vi "PH_Stepmotor_BaseClass.PC set Position.vi"(0 "i ref in":refnum<vi>, 1 "axis":i32=-1, 2 "Position to set":i32, 3 "Set?":bool, 5 "error in (no error)":errorcluster) -> (14 "i ref out":refnum<vi>, 16 "ok?":bool, 19 "error out":errorcluster)   [LabVIEW 2014, in "PH_Stepmotor_BaseClass.lvlib"]
doc: "This VI stores the position in own attributes and sets a flag."
uses:
  PH_Stepmotor_BaseClass.lvlib
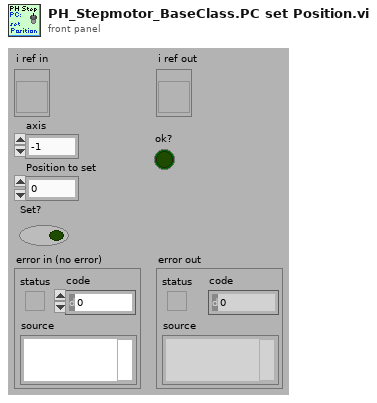
[diagram p1: front panel]
types:
  T1 = typedef "PH_Stepmotor_BaseClass.lvlib/PH_Stepmotor_BaseClass.Axis Attributes.ctl" = cluster{"Settings":T2, "Endswitch?":bool, "DIM Service IDs":T4, "Activity":T5, "Configured?":bool, "Position":cluster{"Current":i32, "Target":i32}, "Position to set":cluster{"New?":bool, "Wanted":i32}, "Stop?":bool, "Reset?":bool, "Move?":bool, "Nothing connected?":bool}
  T2 = typedef "PH_Stepmotor_BaseClass.lvlib/PH_Stepmotor_BaseClass.Axis Settings.ctl" = cluster{"Sign change":bool, "Width":dbl, "Calibration":dbl, "Unit":string, "Motor Type":T3, "Unit Width":string, "Unit CF":string}
  T3 = typedef "PH_Stepmotor_BaseClass.lvlib/PH_Stepmotor_BaseClass.Motor Type.ctl" = enum16{"Unspecific", "OWIS 49.120.2633", "OWIS 49.060.1033", "OWIS 43.040.2558", "Diamond Motion 2200 series", "OWIS 49.120.266B.MV6", "Calorimeter", "Linear Stage 1", "MICOS VT-80", "MICOS VT-80 S", "Standa Rotstage nt0.95A", "PUF RA 320.200", "PUF RA 800.200", "PUF RA 800.400", "PUF RA 400.50", "1324.nn.800.50", "1324.n9c.800.50", "1324.nn.320.200", "1324.nn.400.200", "1324.nn.800.200", "1324.nn.400.50", "1324.8c9c.800.50", "1324.8c9c.400.200"}
  T4 = typedef "PH_Stepmotor_BaseClass.lvlib/PH_Stepmotor_BaseClass.Axis DIM Service IDs.ctl" = cluster{"Settings":i32, "Information":i32}
  T5 = typedef "PH_Stepmotor_BaseClass.lvlib/PH_Stepmotor_BaseClass.Axis Activity.ctl" = enum16{"No Information", "stopped", "running", "Failure", "Alarm", "stopped at backward ES", "stopped at foreward ES"}
  T6 = typedef "PH_Stepmotor_BaseClass.lvlib/PH_Stepmotor_BaseClass.i attribute.ctl" = cluster{"Device Error":errorcluster, "Axes PSDB Thread":cluster{"Ref":refnum<vi>, "Q-Ref":refnum<queue>, "Data Status":T7}, "Axes":T1[], "Axes PSDB Infos":cluster{"GUI Name":string, "PSDB Instance ID":i32, "PSDB Status Service ID":i32, "Axis":i32, "Class":string}[], "GUI Refs":T8}
  T7 = typedef "PH_PSDBWriter.lvlib/PH_PSDBWriter.Data Status.ctl" = i16
  T8 = typedef "PH_Stepmotor_BaseClass.lvlib/PH_Stepmotor_BaseClass.GUI Refs.ctl" = cluster{"Axes Configuration":refnum<vi>, "Device Error":refnum<vi>, "Axes PSDB Infos":refnum<vi>}
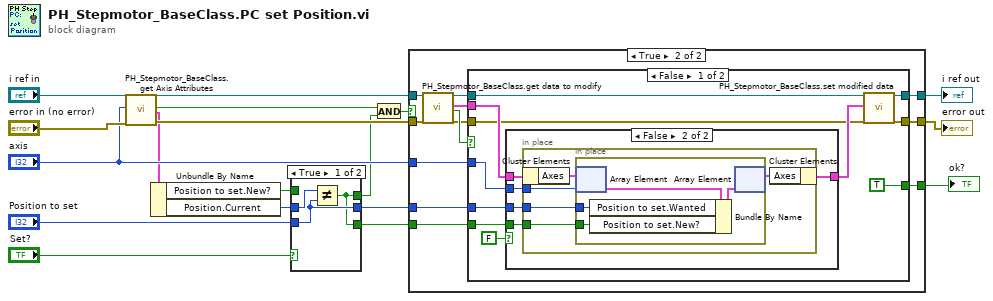
[diagram p0: block diagram]
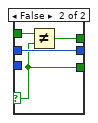
[diagram p2: hidden frame]
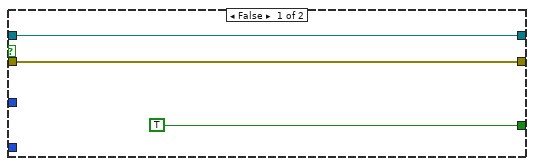
[diagram p3: hidden frame]
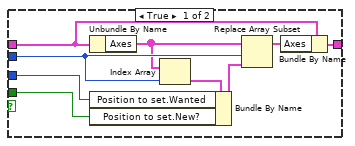
[diagram p4: hidden frame]
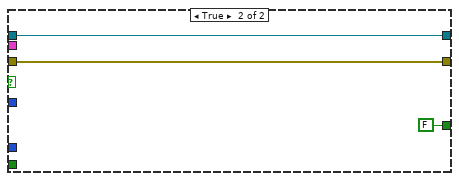
[diagram p5: hidden frame]
diagram:
  n1 = call "PH_Stepmotor_BaseClass.get Axis Attributes.vi"("VI in"="i ref in", "Axis"="axis", "error in (no error)"="error in (no error)") -> ("VI out"=w13:refnum<vi>, "Axis found?"=w11:bool, "Axis Attributes"=w8:T1, "error out"=w15:errorcluster)  [unwired: 13 in]
  n2 = Unbundle By Name(w8) -> ("Position to set.New?"=w3:bool, "Position.Current"=w7:i32)
  n3 = case shown="True" "Set?" {
    selector: "Set?" -> [_ w22]
    tunnel: [w19 w24] -> w2
    tunnel: "Position to set" -> [w20 _]
    tunnel: w7 -> [w21 w23]
    tunnel: [w20 w23] -> w5
    tunnel: w3 -> [_ w25]
    tunnel: [w19 w22] -> w1
    frame True {
      n4 = Not Equal?(x=w21, y=w20) -> (x != y?=w19:bool)
    }
    frame False {
      n5 = Not Equal?(x=w25, y=w22) -> (x != y?=w24:bool)
    }
  }
  n6 = And(x=w11, y=w2) -> (x .and. y?=w10:bool)
  n7 = case shown="True" w10 {
    tunnel: [w28 w36] -> w17
    tunnel: [w27 w35] -> w16
    tunnel: w15 -> [w27 w34]
    tunnel: w13 -> [w28 w33]
    tunnel: "axis" -> [_ w32]
    tunnel: w5 -> [_ w31]
    tunnel: w1 -> [_ w30]
    tunnel: [TRUE w29] -> w4
    frame False {
    }
    frame True {
      n8 = call "PH_Stepmotor_BaseClass.get data to modify.vi"("i ref in"=w33, "error in (no error)"=w34) -> ("i ref out"=w38:refnum<vi>, "i attribute"=w37:T6, "timed out"=w40:bool, "error out"=w39:errorcluster)  [unwired: 14 in]
      n9 = case shown="False" w40 {
        tunnel: [w51 w77] -> w35
        tunnel: w39 -> [w44 w77]
        tunnel: [w50 w76] -> w36
        tunnel: w38 -> [w47 w76]
        tunnel: w37 -> [w49 _]
        tunnel: w32 -> [w46 _]
        tunnel: w31 -> [w45 _]
        tunnel: w30 -> [w42 _]
        tunnel: [TRUE FALSE] -> w29
        frame False {
          n10 = case shown="False" FALSE {
            tunnel: w49 -> [w53 w62]
            tunnel: [w60 w61] -> w48
            tunnel: w46 -> [w58 w65]
            tunnel: w45 -> [w57 w64]
            tunnel: w42 -> [w52 w63]
            frame True {
              n11 = Unbundle By Name(w53) -> ("Axes"=w55:T1[])
              n12 = Index Array(array=w55, index=w58) -> (element=w54:T1)
              n13 = Bundle By Name(cluster=w54, "Position to set.Wanted"=w57, "Position to set.New?"=w52) -> (w56:T1)
              n14 = Replace Array Subset(array=w55, new element=w56, index=w58) -> (w59:T1[])
              n15 = Bundle By Name(cluster=w53, "Axes"=w59) -> (w60:T6)
            }
            frame False {
              n16 = in-place {
                in-place-border: w65 -> [w70]
                in-place-border: w64 -> [w69]
                in-place-border: w63 -> [w68]
                n17 = in-place-cluster #1(w62) -> ("Axes"=w67:T1[])
                n18 = in-place {
                  in-place-border: w69 -> [w72]
                  in-place-border: w68 -> [w71]
                  n19 = in-place-array #2(w67, w70) -> (w74:T1)
                  n20 = Bundle By Name(cluster=w74, "Position to set.Wanted"=w72, "Position to set.New?"=w71) -> (w73:T1)
                  n21 = in-place-array #2(w73) -> (w66:T1[])  [unwired: 1 out]
                }
                n22 = in-place-cluster #1("Axes"=w66) -> (w61:T6)
              }
            }
          }
          n23 = call "PH_Stepmotor_BaseClass.set modified data.vi"("i ref in"=w47, "i attribute"=w48, "error in (no error)"=w44) -> ("i ref out"=w50:refnum<vi>, "error out"=w51:errorcluster)  [unwired: 15 in]
        }
        frame True {
          (unwired) TRUE
        }
      }
    }
  }
  "error out" <- w16
  "i ref out" <- w17
  "ok?" <- w4
